vi "ParseFIFODbl.vi"(1 "photoncount":u32[](array[numeric]), 2 "SPC Format":u16(ring)=2 items=["SPC 630 - 32 bit", "SPC 630 - 48 bit", "SPC 830 - 32 bit", "SPC 130 - 32 bit", ""], 3 "FIFO rawdata":u16[][](array[numeric])) -> (0 "rawdata":T1 {"gap times" format="%.2f"; "invalid times" format="%.2f"; "macro times" format="%.2f"})   [LabVIEW 2009]
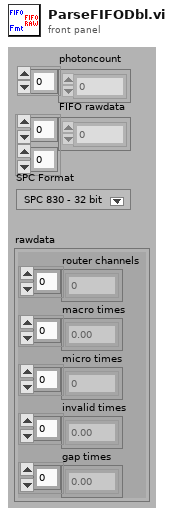
[diagram p1: front panel]
types:
  T1 = cluster{"router channels":u8[], "macro times":dbl[], "micro times":u16[], "invalid times":dbl[], "gap times":dbl[]}
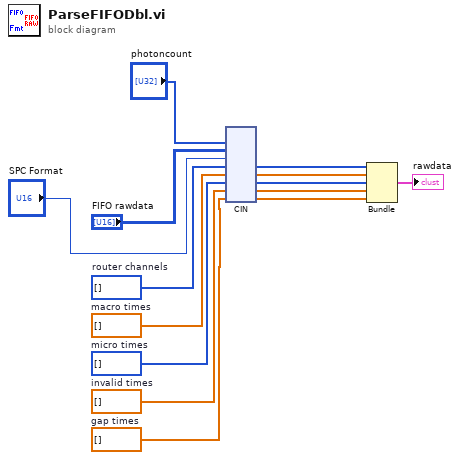
[diagram p0: block diagram]
diagram:
  w6 = dbl[] []  # gap times
  w7 = dbl[] []  # invalid times
  w8 = u16[] []  # micro times
  w9 = dbl[] []  # macro times
  w10 = u8[] []  # router channels
  n1 = cin("photoncount", "FIFO rawdata", "SPC Format", w10, w9, w8, w7, w6) -> (w1:u8[], w2:dbl[], w3:u16[], w4:dbl[], w5:dbl[])  [unwired: 3 in]
  n2 = Bundle("router channels"=w1, "macro times"=w2, "micro times"=w3, "invalid times"=w4, "gap times"=w5) -> (→"rawdata":T1)  [unwired: 1 in]
